vi "Publisher Do.vi"(8 "error in (no error)":errorcluster, 10 "Publisher in":refnum<class "Publisher.lvclass">, 11 "Subscribe Msg":refnum<class "Addressed Msg.lvclass">) -> (0 "error out":errorcluster, 2 "Publisher out":refnum<class "Publisher.lvclass">)   [LabVIEW 2020, in "Publisher.lvlib" / "Addressed Msg.lvclass"]
doc: "This VI delivers the message to the actor by calling the appropriate method(s) on the actor.\n\nThe message is dropped if the forwarding failed."
uses:
  Addressed Msg.lvclass
  C:/Current projects/WS/Framework/Framework/Actors/Publisher/Publisher Messages/Sender Msg/Sender Msg.lvclass
  C:/Current projects/WS/Framework/Framework/Actors/Publisher/Publisher Messages/Publisher Msg/Publisher Msg.lvclass
  Publisher/Publisher.lvclass
  Sender Msg/Sender Msg.lvclass/Sender Msg.ctl
  Publisher Msg/Publisher Msg.lvclass/Publisher Msg.ctl
  Addressed Msg.lvclass/Addressed Msg.ctl
  PPL/HDH.Actor Framework.Core.Actor.lvlibp/1abvi3w/vi.lib/ActorFramework/Message/Message.lvclass
  Publisher Msg/Publisher Msg.lvclass
  Sender Msg/Sender Msg.lvclass
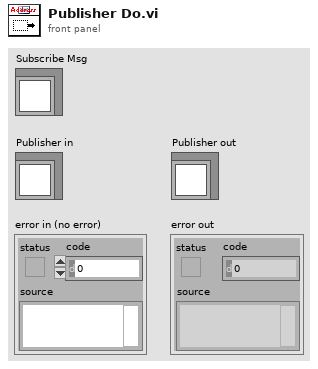
[diagram p1: front panel]
types:
  T1 = typedef "HDH.Actor Framework.Core.Actor.lvlibp/Message Enqueuer.lvclass/Message Priority.ctl" = enum16{"Low", "Normal", "High"}
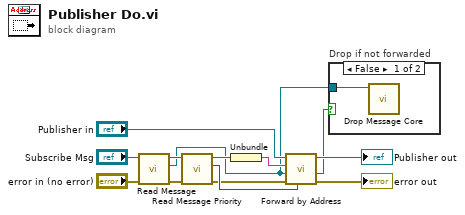
[diagram p0: block diagram]
diagram:
  n1 = call "Read Message.vi"("error in (no error)"="error in (no error)", "Sender Msg in"="Subscribe Msg") -> ("error out"=w4:errorcluster, "Message"=w1:refnum<class "Message.lvclass">, "Sender Msg out"=w2:refnum<class "Addressed Msg.lvclass">)  [unwired: 7 in]
  n2 = call "Read Message Priority.vi"("error in (no error)"=w4, "Publisher Msg in"=w2) -> ("error out"=w10:errorcluster, "Message Priority"=w11:T1, "Publisher Msg out"=w12:refnum<class "Addressed Msg.lvclass">)  [unwired: 7 in]
  n3 = Unbundle(w12) -> (w5:string)
  n4 = call "Forward by Address.vi"("Message Priority (Normal)"=w11, "error in (no error)"=w10, "Message"=w1, "Target Enqueuer ID"=w5, "Publisher in"="Publisher in") -> ("error out"=→"error out":errorcluster, "Message forwarded?"=w7:bool, "Publisher out"=→"Publisher out":refnum<class "Publisher.lvclass">)  [unwired: 4 in]
  n5 = case "Drop if not forwarded" shown="False" w7 {
    tunnel: w1 -> [w14 _]
    frame False {
      n6 = call-dynamic "Drop Message Core.vi"("Message in"=w14) -> ()  [unwired: 11 in]
    }
    frame True {
    }
  }
